vi "cw2.vi"() -> ()   [LabVIEW 2017]
panel:
  in  "Temperature in":bool
  out "y":dbl
  in  "Knob":u8(knob) scale=0.0..1.0
  in  "Przekroczenie zakresu":bool
  out "Resistance Chart":dbl(graph)
  in  "R or T":u32(knob) scale=0.0..1.0
  out "Temperature Chart":dbl(graph)
  out "Temperature":string
  out "Przekroczenie":bool
  out "error out":errorcluster
  in  "Precision":dbl
  out "Result in Ohm":dbl
  in  "seconds to wait":dbl=10.0 min=0.5 max=10.0 step=0.5
  in  "stop":bool
  out "Convert from":string
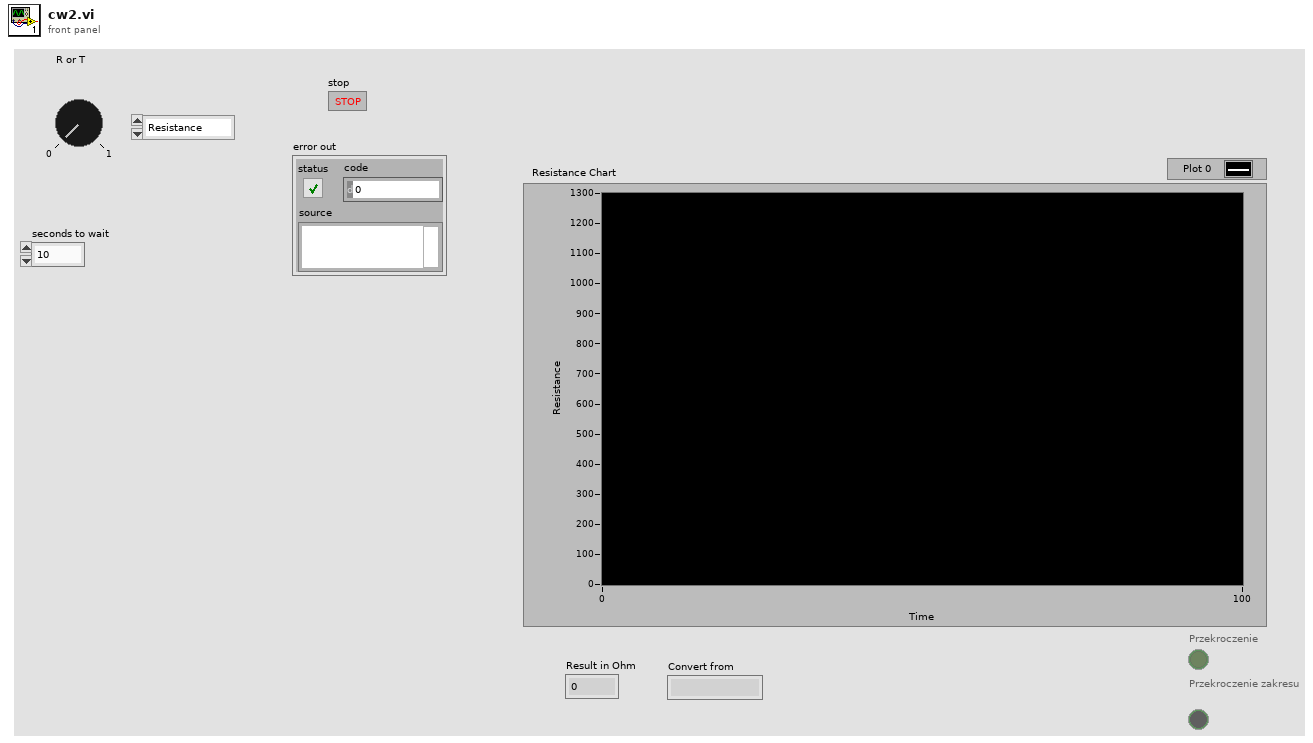
[diagram p1: front panel]
types:
  T1 = enum8{"Enabled", "Disabled", "Disabled and Grayed Out"}
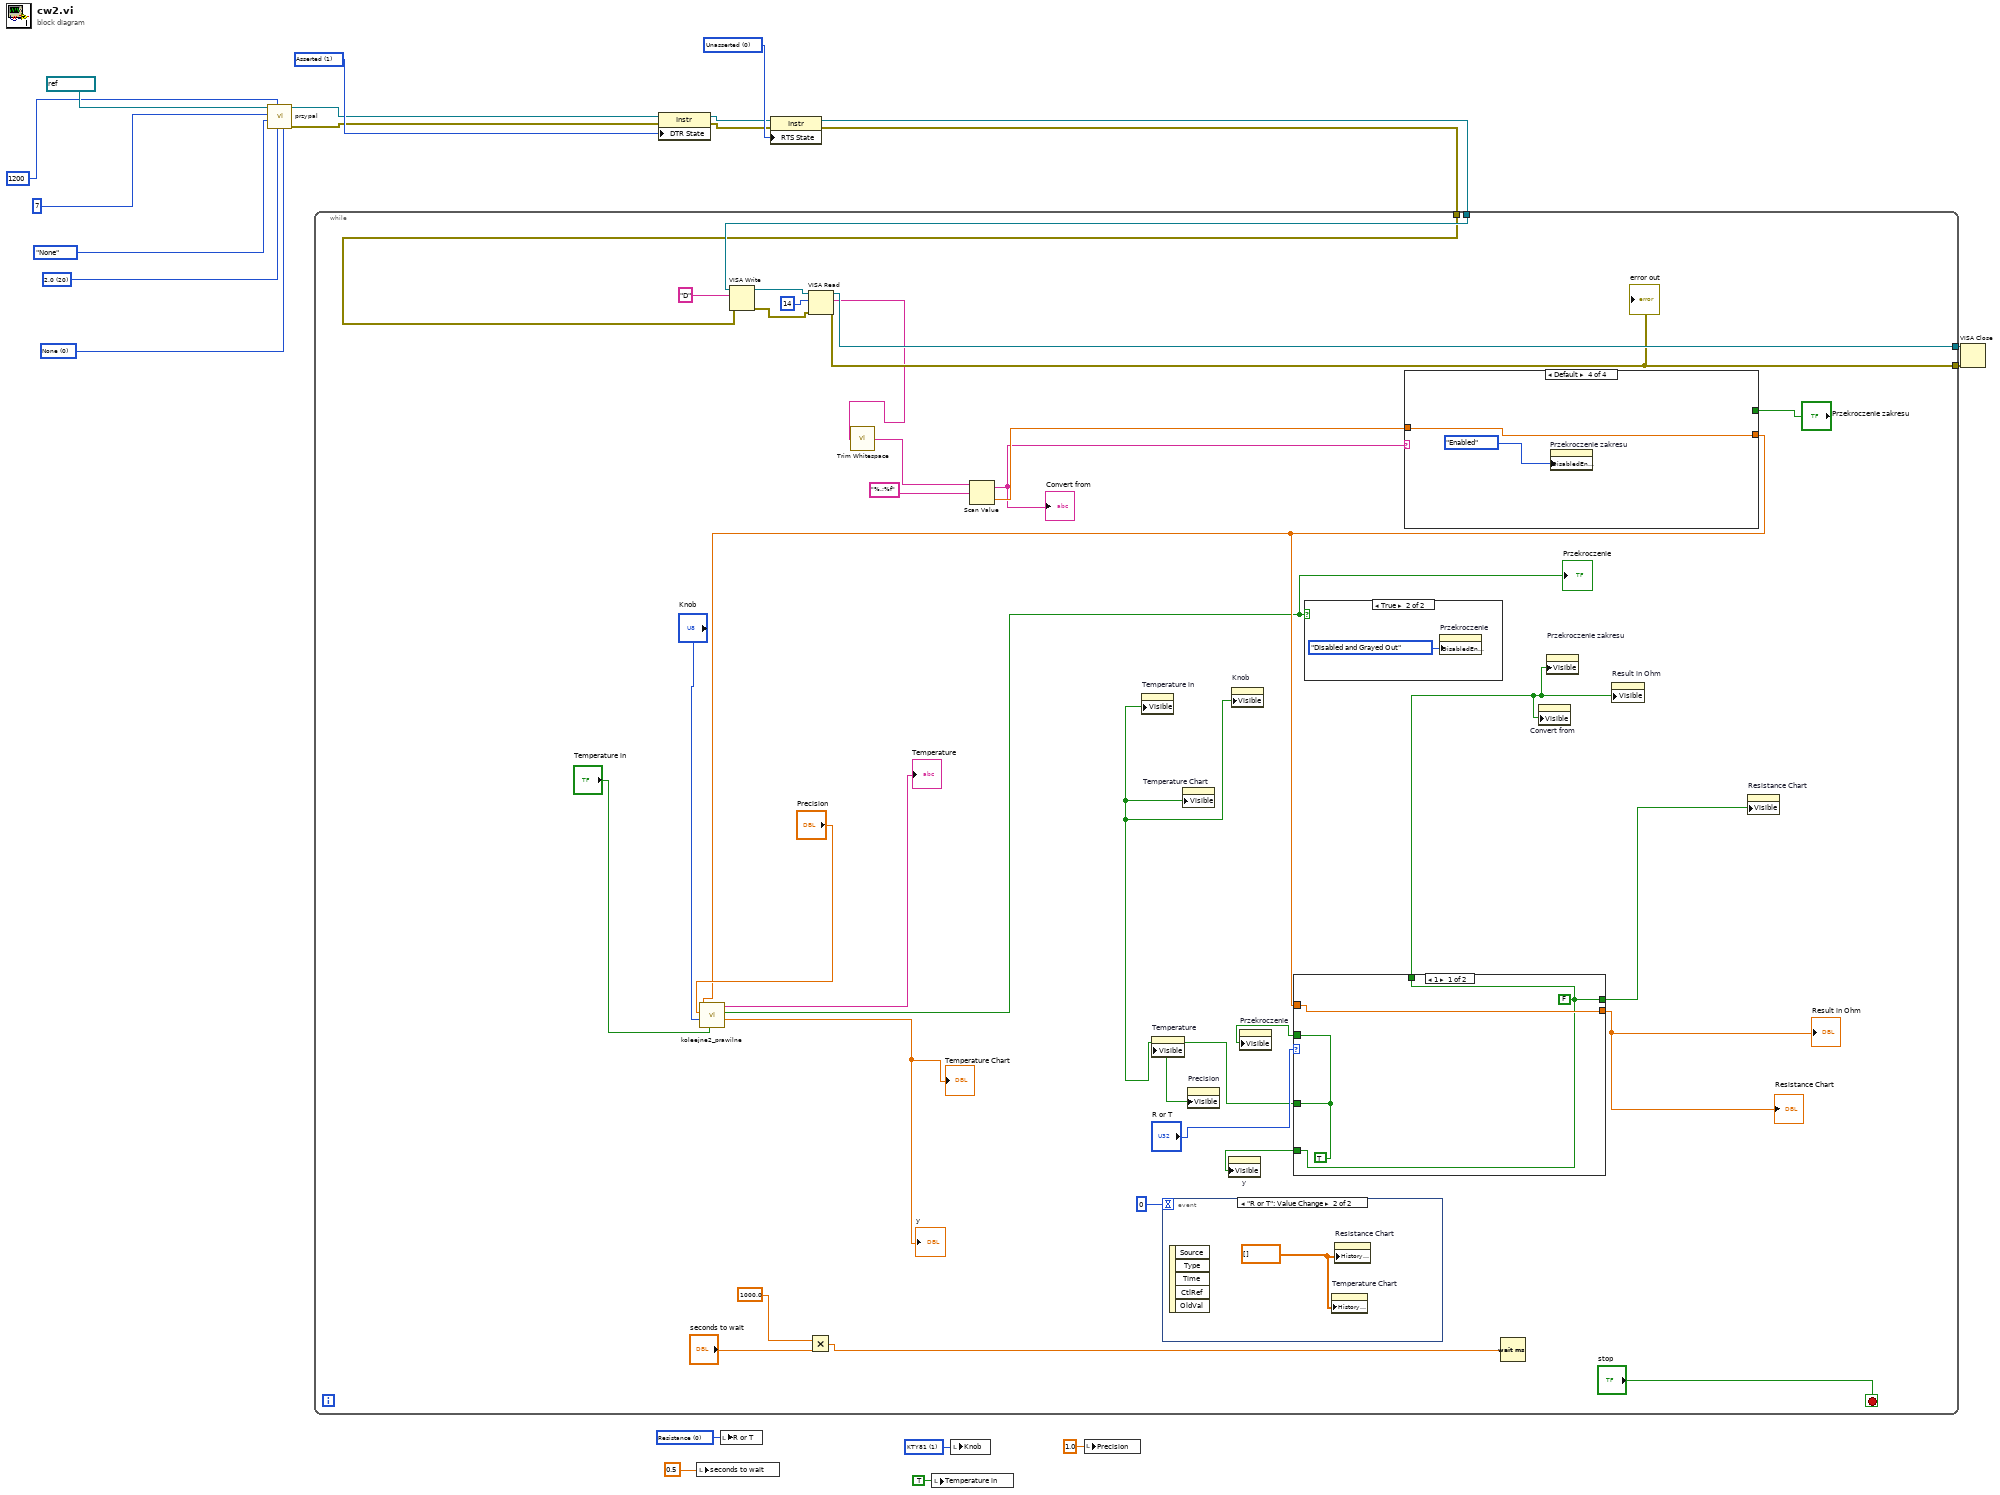
[diagram p0: block diagram]
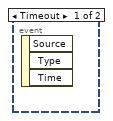
[diagram p2: hidden frame]
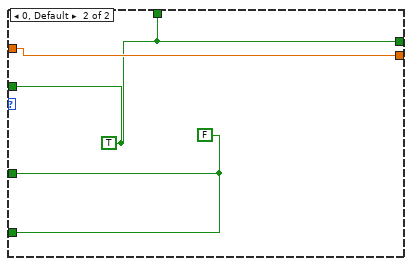
[diagram p3: hidden frame]
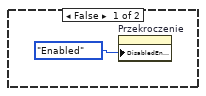
[diagram p4: hidden frame]
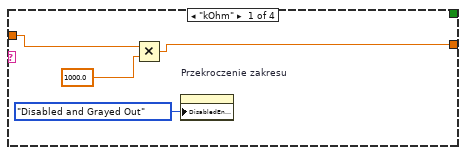
[diagram p5: hidden frame]
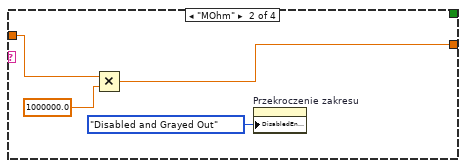
[diagram p6: hidden frame]
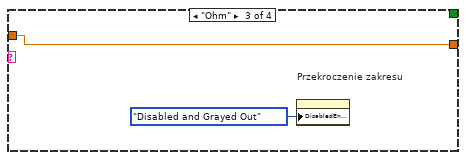
[diagram p7: hidden frame]
diagram:
  w2 = u8 1 items=["Pt100", "KTY81"] ("Knob")
  w4 = u32 0 items=["Resistance", "Temperature"] ("R or T")
  w14 = i16 0 items=["Unknown"=-1, "Unasserted"=0, "Asserted"=1] ("Serial Settings:Modem Line Settings:Line RTS State")
  w15 = i16 1 items=["Unknown"=-1, "Unasserted"=0, "Asserted"=1] ("Serial Settings:Modem Line Settings:Line DTR State")
  w16 = u16 0 items=["None", "XON/XOFF", "RTS/CTS", "XON/XOFF & RTS/CTS", "DTR/DSR", "XON/XOFF & DTR/DSR"] ("flow control (0:none)")
  w21 = u16 20 items=["1.0"=10, "1.5"=15, "2.0"=20] ("stop bits (10: 1 bit)")
  n1 = call "przypal.vi"("flow control (0:none)"=w16, "stop bits (10: 1 bit)"=w21, "baud rate (9600)"=u32 1200, "parity (0:none)"=enum16{"None", "Odd", "Even", "Mark", "Space"}."None", "data bits (8)"=u16 7, "VISA Refnum in"=refnum<visa-resource-name> "COM1" ("VISA resource name")) -> ("error out"=w10:errorcluster, "VISA Refnum out"=w11:refnum<visa-resource-name>)  [unwired: 4 in]
  n2 = property class="Instr"(reference=w11, error in=w10, "DTR State"=w15) -> (reference out=w13:refnum<visa-resource-name>, error out=w12:errorcluster)
  n3 = local write "seconds to wait"(0.5 ("milliseconds to wait")) -> ()
  n4 = local write "R or T"(w4) -> ()
  n5 = property class="Instr"(reference=w13, error in=w12, "RTS State"=w14) -> (reference out=w9:refnum<visa-resource-name>, error out=w8:errorcluster)
  n6 = while {
    tunnel: w9 -> [w53]
    tunnel: w8 -> [w52]
    tunnel: [w44] -> w7
    tunnel: [w43] -> w6
    stop <- "stop" stop-if-true
    n7 = VISA Write(VISA resource name=w53, write buffer="D", error in (no error)=w52) -> (VISA resource name out=w46:refnum<visa-resource-name>, error out=w45:errorcluster)  [unwired: 1 out]
    n8 = Multiply(x=1000.0, y="seconds to wait") -> (x*y=w48:dbl)
    n9 = VISA Read(VISA resource name=w46, byte count=u32 14, error in (no error)=w45) -> (VISA resource name out=w44:refnum<visa-resource-name>, read buffer=w33:string, error out=w43:errorcluster)  [unwired: 1 out]
    "error out" <- w43
    n10 = call <vilib>:"Trim Whitespace.vi"("string"=w33) -> ("trimmed string"=w41:string)  [unwired: 1 in]
    n11 = Scan Value(string=w41, format string="%.;%f") -> (output string=w32:string, value=w40:dbl)  [unwired: 1 in]
    "Convert from" <- w32
    n12 = event shown="[1] \"R or T\": Value Change" {
      selector: _ -> [_ _]
      dyn-events: _ -> [_ _]
      timeout: 0 -> [_ _]
      event Timeout {
        n13 = event-data() -> ()  [unwired: 1 in, 3 out]
      }
      event "R or T": Value Change {
        w55 = dbl[] [] ("History Data")
        n14 = event-data() -> ()  [unwired: 1 in, 5 out]
        n15 = property on="Temperature Chart" class="WFChart (strict)"("History Data"=w55) -> ()  [unwired: 2 in, 2 out]
        n16 = property on="Resistance Chart" class="WFChart (strict)"("History Data"=w55) -> ()  [unwired: 2 in, 2 out]
      }
    }
    n17 = case shown="Default" w32 {
      tunnel: w40 -> [w66 w71 w73 w74]
      tunnel: [w65 w70 w73 w74] -> w27
      tunnel: "Przekroczenie zakresu" -> [_ _ _ _]
      frame "kOhm" {
        n18 = Multiply(x=w66, y=1000.0) -> (x*y=w65:dbl)
        n19 = property on="Przekroczenie zakresu" class="Bool (strict)"("DisabledEnum"=T1."Disabled and Grayed Out" ("Disabled")) -> ()  [unwired: 2 in, 2 out]
      }
      frame "MOhm" {
        n20 = Multiply(x=w71, y=1000000.0) -> (x*y=w70:dbl)
        n21 = property on="Przekroczenie zakresu" class="Bool (strict)"("DisabledEnum"=T1."Disabled and Grayed Out" ("Disabled")) -> ()  [unwired: 2 in, 2 out]
      }
      frame "Ohm" {
        n22 = property on="Przekroczenie zakresu" class="Bool (strict)"("DisabledEnum"=T1."Disabled and Grayed Out" ("Disabled")) -> ()  [unwired: 2 in, 2 out]
      }
      frame Default {
        n23 = property on="Przekroczenie zakresu" class="Bool (strict)"("DisabledEnum"=T1."Enabled" ("Disabled")) -> ()  [unwired: 2 in, 2 out]
      }
    }
    n24 = call "koleejne2_prawilne.vi"("Temperature in"="Temperature in", "Knob"="Knob", "Precision"="Precision", "Numeric"=w27) -> ("y"=→"Temperature Chart" →"y":dbl, "Boolean"=w26:bool, "String"=→"Temperature":string)  [unwired: 5 in]
    "Przekroczenie" <- w26
    n25 = case shown="1" "R or T" {
      tunnel: w27 -> [w58 w61]
      tunnel: [w58 w61] -> w38
      tunnel: [w56 w60] -> w34
      tunnel: [w57 w59] -> w23
      tunnel: [w56 w60] -> w37
      tunnel: [w57 w60] -> w36
      tunnel: [w56 w59] -> w22
      frame 1 {
        w56 = FALSE
        w57 = TRUE
      }
      frame 0, Default {
        w59 = FALSE
        w60 = TRUE
      }
    }
    "Result in Ohm" <- w38
    "Resistance Chart" <- w38
    n26 = property on="Temperature in" class="Bool (strict)"("Visible"=w23) -> ()  [unwired: 2 in, 2 out]
    n27 = property on="Temperature" class="Str"("Visible"=w23) -> ()  [unwired: 2 in, 2 out]
    n28 = property on="Temperature Chart" class="WFChart (strict)"("Visible"=w23) -> ()  [unwired: 2 in, 2 out]
    n29 = property on="Precision" class="DigNum (strict)"("Visible"=w23) -> ()  [unwired: 2 in, 2 out]
    n30 = property on="y" class="DigNum (strict)"("Visible"=w22) -> ()  [unwired: 2 in, 2 out]
    n31 = property on="Knob" class="Knob (strict)"("Visible"=w23) -> ()  [unwired: 2 in, 2 out]
    n32 = property on="Przekroczenie" class="Bool (strict)"("Visible"=w36) -> ()  [unwired: 2 in, 2 out]
    n33 = case shown="True" w26 {
      frame False {
        n34 = property on="Przekroczenie" class="Bool (strict)"("DisabledEnum"=T1."Enabled" ("Disabled")) -> ()  [unwired: 2 in, 2 out]
      }
      frame True {
        n35 = property on="Przekroczenie" class="Bool (strict)"("DisabledEnum"=T1."Disabled and Grayed Out" ("Disabled")) -> ()  [unwired: 2 in, 2 out]
      }
    }
    n36 = Wait (ms)(milliseconds to wait=w48) -> ()  [unwired: 1 out]
    n37 = property on="Convert from" class="Str"("Visible"=w34) -> ()  [unwired: 2 in, 2 out]
    n38 = property on="Przekroczenie zakresu" class="Bool (strict)"("Visible"=w34) -> ()  [unwired: 2 in, 2 out]
    n39 = property on="Result in Ohm" class="DigNum (strict)"("Visible"=w34) -> ()  [unwired: 2 in, 2 out]
    n40 = property on="Resistance Chart" class="WFChart (strict)"("Visible"=w37) -> ()  [unwired: 2 in, 2 out]
  }
  n41 = local write "Temperature in"(TRUE ("Temperature in")) -> ()
  n42 = local write "Knob"(w2) -> ()
  n43 = local write "Precision"(1.0 ("Precision")) -> ()
  n44 = VISA Close(VISA resource name=w7, error in (no error)=w6) -> ()  [unwired: 1 out]
